vi "Dropdown - Engine.vi"() -> ()   [LabVIEW 2013]
uses:
  <vilib>/Utility/miscctls.llb/LVRectTypeDef.ctl
panel:
  in  "Ring":u16(ring) items=["", "this", "is", "for", "testing"]
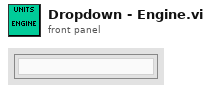
[diagram p1: front panel]
types:
  T1 = enum16{"Set Abbreviations", "Set Engine Mode", "Set Enum Position", "Get Abbreviation", "Write Abbreviation", "Read Enum Position", "Read Engine Mode", "Read Abbreviations", "Engine Started", "Check Engine", "Init Global", "Set Cursor", "Read Cursor"}
  T2 = enum16{"Idle", "Reveal Dropdown", "Hide FP", "Set Options", "Close Program"}
  T3 = typedef "LVRectTypeDef.ctl" = cluster{"Left":i16, "Top":i16, "Right":i16, "Bottom":i16}
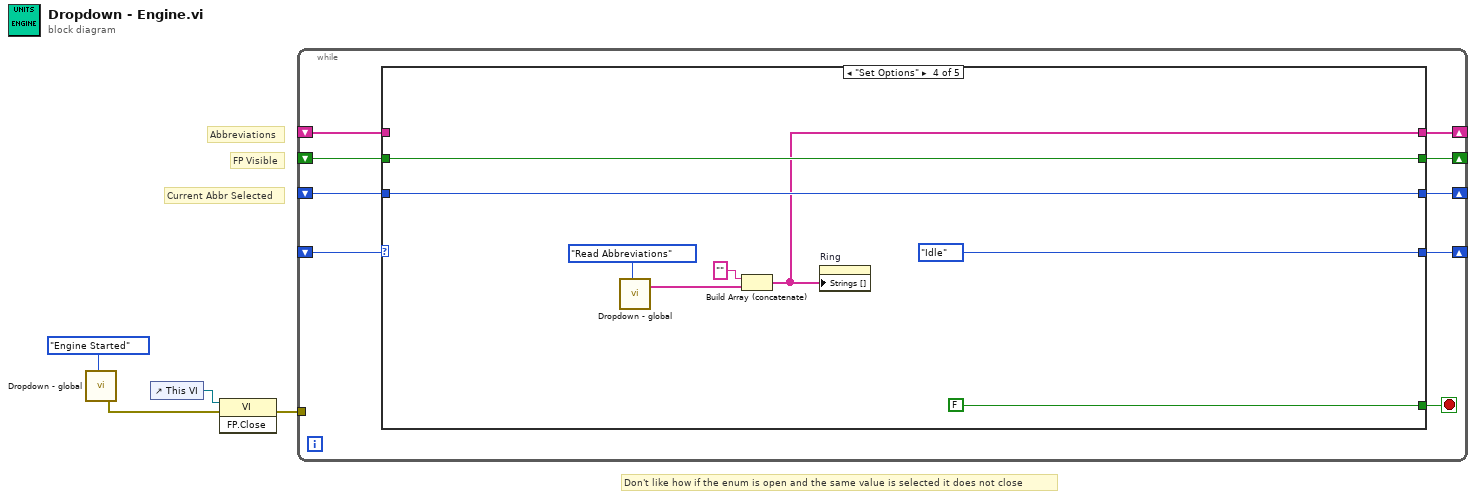
[diagram p0: block diagram]
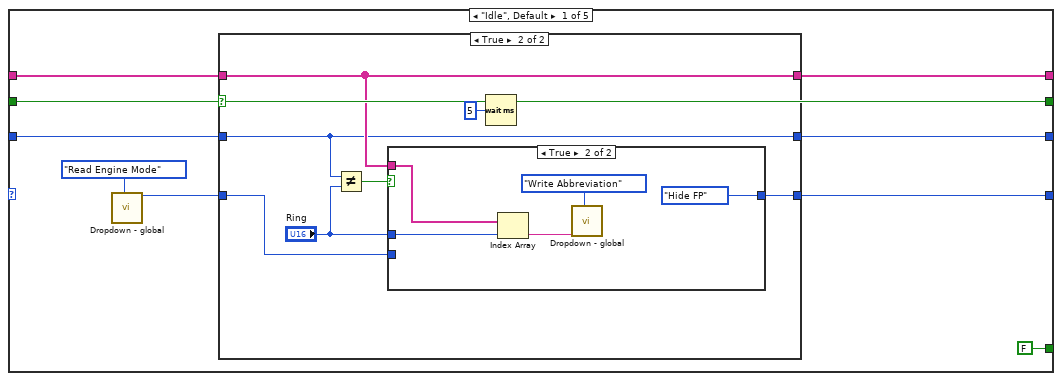
[diagram p2: hidden frame]
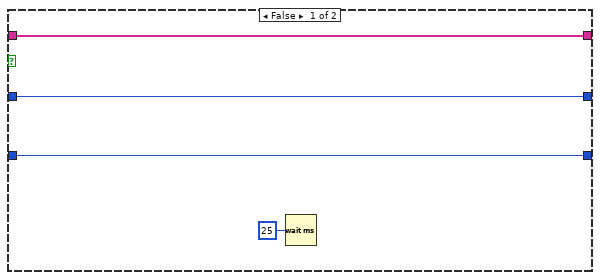
[diagram p3: hidden frame]
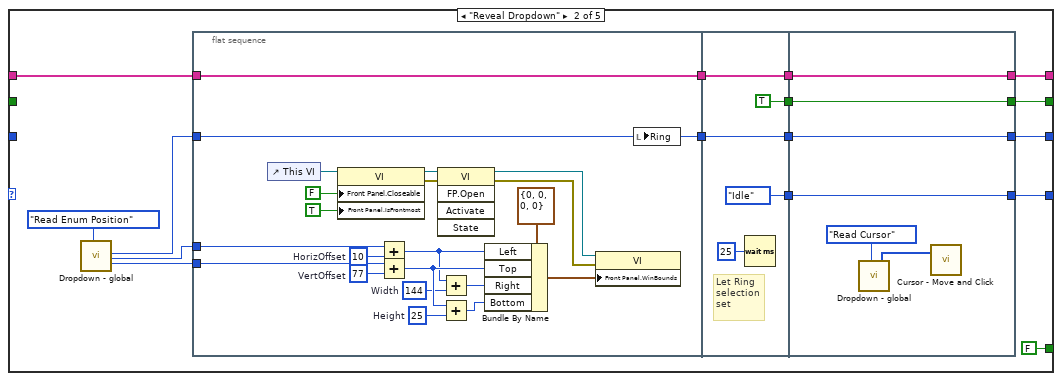
[diagram p5: hidden frame]
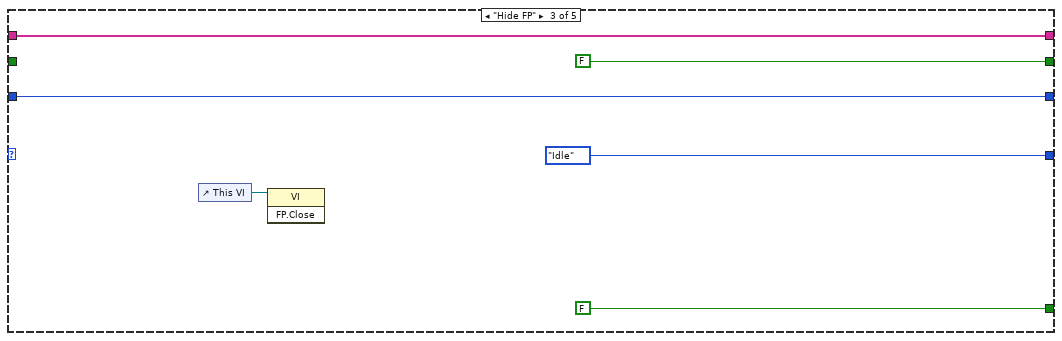
[diagram p6: hidden frame]
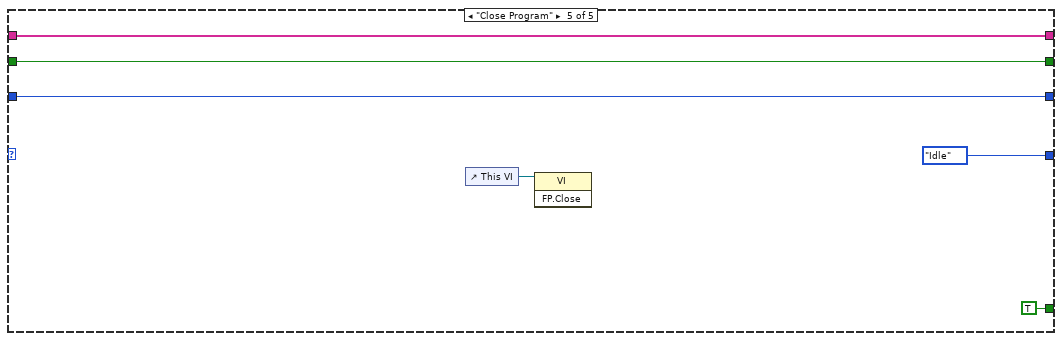
[diagram p7: hidden frame]
diagram:
  # "Don't like how if the enum is open and the same value is selected it does not close"
  # "Current Abbr Selected"
  # "FP Visible"
  # "Abbreviations"
  n1 = call "Dropdown - global.vi"("Global Mode"=T1."Engine Started") -> ("Error Out"=w3:errorcluster)  [unwired: 10 in, 8 out]
  n2 = control-ref of="This VI"() -> (w4:refnum<vi>)
  n3 = invoke class="VI" method="FP.Close"(reference=w4, error in=w3) -> (error out=w2:errorcluster)  [unwired: 1 in, 2 out]
  n4 = while {
    shift-right: [w13] -> _
    shift-left: _ -> [w12]
    shift-right: [w11] -> _
    shift-left: _ -> [w10]
    shift-right: [w9] -> _
    shift-left: _ -> [w8]
    shift-right: [w7] -> _
    shift-left: _ -> [w6]
    tunnel: w2 -> [_]
    stop <- w5 stop-if-true
    n5 = case shown="\"Set Options\"" w10 {
      tunnel: [w21 w53 w92 w94 w103] -> w13
      tunnel: w12 -> [w22 w54 w92 _ w103]
      tunnel: [w17 w46 T2."Idle" ("Mode") T2."Idle" ("Mode") T2."Idle" ("Mode")] -> w11
      tunnel: [w20 w52 FALSE w101 w104] -> w9
      tunnel: w8 -> [w20 _ _ w101 w104]
      tunnel: [w19 w51 w91 w99 w105] -> w7
      tunnel: w6 -> [w18 _ w91 w99 w105]
      tunnel: [FALSE FALSE FALSE FALSE TRUE] -> w5
      frame "Idle", Default {
        n6 = call "Dropdown - global.vi"("Global Mode"=T1."Read Engine Mode") -> ("Engine Mode Out"=w16:T2)  [unwired: 10 in, 8 out]
        n7 = case shown="True" w20 {
          tunnel: w22 -> [w25 w33]
          tunnel: [w25 w33] -> w21
          tunnel: [w24 w32] -> w19
          tunnel: w18 -> [w24 w32]
          tunnel: w16 -> [w23 w28]
          tunnel: [w23 w27] -> w17
          frame False {
            n8 = Wait (ms)(milliseconds to wait=u32 25) -> ()  [unwired: 1 out]
          }
          frame True {
            n9 = Not Equal?(x=w32, y="Ring") -> (x != y?=w29:bool)
            n10 = case shown="True" w29 {
              tunnel: "Ring" -> [_ w39]
              tunnel: w33 -> [_ w38]
              tunnel: w28 -> [w34 _]
              tunnel: [w34 T2."Hide FP" ("Mode")] -> w27
              frame False {
              }
              frame True {
                n11 = Index Array(array=w38, index=w39) -> (element=w37:string)
                n12 = call "Dropdown - global.vi"("Abbr In"=w37, "Global Mode"=T1."Write Abbreviation") -> ()  [unwired: 9 in, 9 out]
              }
            }
            n13 = Wait (ms)(milliseconds to wait=u32 5) -> ()  [unwired: 1 out]
          }
        }
      }
      frame "Reveal Dropdown" {
        n14 = call "Dropdown - global.vi"("Global Mode"=T1."Read Enum Position") -> ("Ring Index Out"=w47:u16, "Left Out"=w50:i16, "Top Out"=w49:i16)  [unwired: 10 in, 6 out]
        n15 = flat-sequence {
          tunnel: [w65] -> w55
          tunnel: w54 -> [w65]
          tunnel: w50 -> [w64]
          tunnel: w49 -> [w63]
          tunnel: [w58] -> w48
          tunnel: w47 -> [w58]
          tunnel: w55 -> [w81]
          tunnel: w48 -> [w79]
          tunnel: [w81] -> w45
          tunnel: [TRUE] -> w44
          tunnel: [w79] -> w43
          tunnel: [T2."Idle" ("Mode")] -> w42
          tunnel: [w84] -> w46
          tunnel: [w85] -> w51
          tunnel: [w86] -> w52
          tunnel: [w87] -> w53
          tunnel: w45 -> [w87]
          tunnel: w44 -> [w86]
          tunnel: w43 -> [w85]
          tunnel: w42 -> [w84]
          frame #0 {
            w73 = i16 77  # VertOffset
            w72 = i16 10  # HorizOffset
            w69 = i16 144  # Width
            w68 = i16 25  # Height
            n16 = control-ref of="This VI"() -> (w76:refnum<vi>)
            n17 = property class="VI"(reference=w76, "Front Panel.Closeable"=FALSE ("Front Panel Window:Closeable"), "Front Panel.IsFrontmost"=TRUE ("Front Panel Window:Is Frontmost")) -> (reference out=w60:refnum<vi>, error out=w62:errorcluster)  [unwired: 1 in]
            n18 = Add(x=w64, y=w72) -> (x+y=w70:i16)
            n19 = Add(x=w63, y=w73) -> (x+y=w71:i16)
            n20 = invoke class="VI" method="FP.Open"(reference=w60, error in=w62) -> (reference out=w59:refnum<vi>, error out=w61:errorcluster)  [unwired: 3 in, 3 out]
            n21 = Add(x=w70, y=w69) -> (x+y=w57:i16)
            n22 = Add(x=w71, y=w68) -> (x+y=w56:i16)
            n23 = Bundle By Name(cluster=T3 {"Left"=0, "Top"=0, "Right"=0, "Bottom"=0} ("Front Panel Window:Window Bounds"), "Left"=w70, "Top"=w71, "Right"=w57, "Bottom"=w56) -> (w66:T3)
            n24 = property class="VI"(reference=w59, error in=w61, "Front Panel.WinBounds"=w66) -> ()  [unwired: 2 out]
            n25 = local write "Ring"(w58) -> ()
          }
          frame #1 {
            # "Let Ring\nselection\nset"
            n26 = Wait (ms)(milliseconds to wait=u32 25) -> ()  [unwired: 1 out]
          }
          frame #2 {
            n27 = call "Dropdown - global.vi"("Global Mode"=T1."Read Cursor") -> ("Cursor Pos Out"=w83:i32[])  [unwired: 10 in, 8 out]
            n28 = call "Cursor - Move and Click.vi"("Cursor Position - Write"=w83) -> ()  [unwired: 3 in]
          }
        }
      }
      frame "Hide FP" {
        n29 = control-ref of="This VI"() -> (w90:refnum<vi>)
        n30 = invoke class="VI" method="FP.Close"(reference=w90) -> ()  [unwired: 2 in, 3 out]
      }
      frame "Set Options" {
        n31 = call "Dropdown - global.vi"("Global Mode"=T1."Read Abbreviations") -> ("AbbrS Out"=w95:string[])  [unwired: 10 in, 8 out]
        n32 = Build Array (concatenate)("", w95) -> (w94:string[])
        n33 = property on="Ring" class="Ring (strict)"("Strings []"=w94) -> ()  [unwired: 2 in, 2 out]
      }
      frame "Close Program" {
        n34 = control-ref of="This VI"() -> (w106:refnum<vi>)
        n35 = invoke class="VI" method="FP.Close"(reference=w106) -> ()  [unwired: 2 in, 3 out]
      }
    }
  }
